vi "AlazarGetBoardKind.vi"(0 "Handle":u64, 1 "error in (no error)":errorcluster) -> (2 "Handle":u64, 3 "Board Kind":u32, 4 "Return Code":u32, 5 "error out":errorcluster)   [LabVIEW 2018]
doc: "Get a board model identifier of the board associated with a board handle."
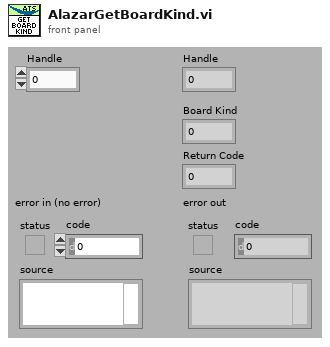
[diagram p1: front panel]
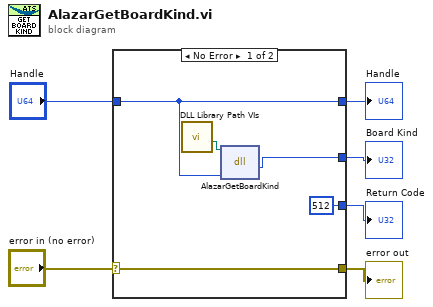
[diagram p0: block diagram]
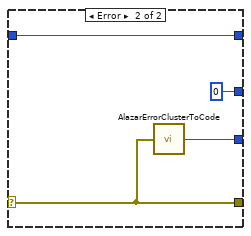
[diagram p2: hidden frame]
diagram:
  n1 = case shown="No Error" "error in (no error)" {
    selector: "error in (no error)" -> [w10 w15]
    tunnel: [w10 w15] -> w5
    tunnel: [512 w14] -> w4
    tunnel: "Handle" -> [w9 w13]
    tunnel: [w9 w13] -> w2
    tunnel: [w8 0] -> w1
    frame No Error {
      n2 = call "DLL Library Path VIs.vi"() -> ("Alazar"=w7:path)  [unwired: 9 in, 2 out]
      n3 = dll-call lib="C:/Project/SerialSectOCT - FFT GPU/SerialSectOCT/Labview Software/DLL/ATSApi.dll" fn="AlazarGetBoardKind"(path in=w7, "handle"=w9) -> ("return type"=w8:u32)  [unwired: 3 in, 2 out]
    }
    frame Error {
      n4 = call "AlazarErrorClusterToCode.vi"("error in (no error)"=w15) -> ("Error Code"=w14:u32)
    }
  }
  "Handle" <- w2
  "error out" <- w5
  "Return Code" <- w4
  "Board Kind" <- w1
